vi "save current settings.vi"(4 "error in":errorcluster, 6 "VNALogOpt":T1={"VNALogSelect"=enum."No Selection", "VNALogTIncr"=5.0, "VNALogTList"=""} {"VNALogTIncr" min=1.0 step=1.0 format="%#.1g"}, 7 "Path":path) -> (0 "error out":errorcluster)   [LabVIEW 2023]
uses:
  controls/VNALogOpt.ctl
  <vilib>/Utility/config.llb/Write Key (Path).vi
  <vilib>/Utility/config.llb/NI_LVConfig.lvlib
  <userlib>/_OpenG.lib/variantconfig/variantconfig.llb/openg_variant_configuration_file.lvlib
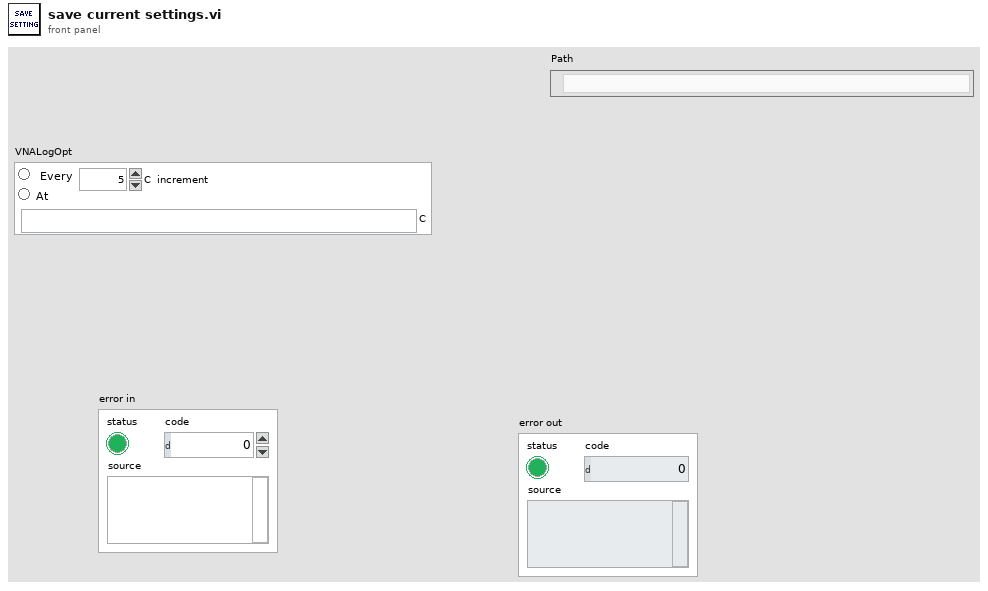
[diagram p1: front panel]
types:
  T1 = typedef "VNALogOpt.ctl" = cluster{"VNALogSelect":enum32{"No Selection", "TempIncr", "TempList"}, "VNALogTIncr":dbl, "VNALogTList":string}
  T2 = typedef "NI_LVConfig.lvlib/Config Data RefNum.ctl" = refnum<k1>
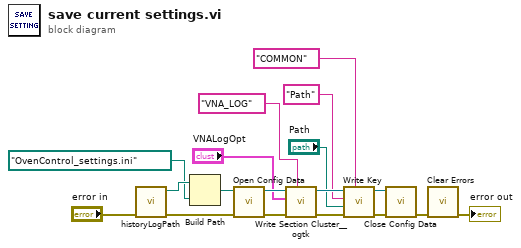
[diagram p0: block diagram]
diagram:
  n1 = call "historyLogPath.vi"("error in"="error in") -> ("error out"=w15:errorcluster, "Path Out"=w18:path)  [unwired: 4 in, 1 out]
  n2 = Build Path(base path=w18, name or relative path=path "OvenControl_settings.ini") -> (appended path=w16:path)
  n3 = call <vilib>:"Open Config Data.vi"("error in (no error)"=w15, "configuration file path"=w16) -> ("error out"=w13:errorcluster, "refnum"=w14:T2)  [unwired: 7 in, 1 out]
  n4 = call <userlib>:"Write Section Cluster__ogtk.vi"("section (optional)"="VNA_LOG", "error in (no error)"=w13, "Section Formatted Cluster"="VNALogOpt", "refnum"=w14) -> ("error out"=w11:errorcluster, "dup refnum"=w9:T2)  [unwired: 6 in]
  n5 = call-poly <vilib>:"Write Key.vi"("section"="COMMON", "error in (no error)"=w11, "value"="Path", "key"="Path", "refnum"=w9) -> ("error out"=w2:errorcluster, "refnum out"=w3:T2)  [unwired: 4 in, 1 out]
  n6 = call <vilib>:"Close Config Data.vi"("error in (no error)"=w2, "refnum"=w3) -> ("error out"=w1:errorcluster)  [unwired: 8 in, 1 out]
  n7 = call <vilib>:"Clear Errors.vi"("error in (no error)"=w1) -> ("error out"=→"error out":errorcluster)  [unwired: 5 in, 1 out]
